vi "对ROI进行分析-修改中.vi"() -> ()   [LabVIEW 2018]
uses:
  <vilib>/vision/NI_Vision_Development_Module.lvlib
panel:
  in  "Pixel Measurements":T1=[0, 1, 2, 3, 42, 8, 9, 10, 11, 4, 5, 6, 7] items=["Center of Mass X", "Center of Mass Y", "First Pixel X", "First Pixel Y", "Bounding Rect Left", "Bounding Rect Top", "Bounding Rect Right", "Bounding Rect Bottom", "Max Feret Diameter Start X", "Max Feret Diameter Start Y", "Max Feret Diameter End X", "Max Feret Diameter End Y", "Max Horiz. Segment Length Left", "Max Horiz. Segment Length Right", "Max Horiz. Segment Length Row", "-", "Bounding Rect Width", "Bounding Rect Height", "Bounding Rect Diagonal", "Perimeter", "Convex Hull Perimeter", "Holes' Perimeter", "Max Feret Diameter", "Equivalent Ellipse Major Axis", "Equivalent Ellipse Minor Axis", "Equivalent Ellipse Minor Axis (Feret)", "Equivalent Rect Long Side", "Equivalent Rect Short Side", "Equivalent Rect Diagonal", "Equivalent Rect Short Side (Feret)", "Average Horiz. Segment Length", "Average Vert. Segment Length", "Hydraulic Radius", "Waddel Disk Diameter", "-", "Area", "Holes' Area", "Particle & Holes' Area", "Convex Hull Area", "Image Area", "-", "Number of Holes", "Number of Horiz. Segments", "Number of Vert. Segments", "-", "Orientation", "Max Feret Diameter Orientation", "-", "% Area/Image Area", "% Area/(Particle & Holes' Area)", "Ratio of Equivalent Ellipse Axes", "Ratio of Equivalent Rect Sides", "-", "Elongation Factor", "Compactness Factor", "Heywood Circularity Factor", "Type Factor", "-", "Sum X", "Sum Y", "Sum XX", "Sum XY", "Sum YY", "Sum XXX", "Sum XXY", "Sum XYY", "Sum YYY", "-", "Moment of Inertia XX", "Moment of Inertia XY", "Moment of Inertia YY", "Moment of Inertia XXX", "Moment of Inertia XXY", "Moment of Inertia XYY", "Moment of Inertia YYY", "Norm. Moment of Inertia XX", "Norm. Moment of Inertia XY", "Norm. Moment of Inertia YY", "Norm. Moment of Inertia XXX", "Norm. Moment of Inertia XXY", "Norm. Moment of Inertia XYY", "Norm. Moment of Inertia YYY", "Hu Moment 1", "Hu Moment 2", "Hu Moment 3", "Hu Moment 4", "Hu Moment 5", "Hu Moment 6", "Hu Moment 7"]
  in  "Selection Values":T3(array[cluster]) {"Measurement Parameter" items=["Center of Mass X", "Center of Mass Y", "First Pixel X", "First Pixel Y", "Bounding Rect Left", "Bounding Rect Top", "Bounding Rect Right", "Bounding Rect Bottom", "Max Feret Diameter Start X", "Max Feret Diameter Start Y", "Max Feret Diameter End X", "Max Feret Diameter End Y", "Max Horiz. Segment Length Left", "Max Horiz. Segment Length Right", "Max Horiz. Segment Length Row", "-", "Bounding Rect Width", "Bounding Rect Height", "Bounding Rect Diagonal", "Perimeter", "Convex Hull Perimeter", "Holes' Perimeter", "Max Feret Diameter", "Equivalent Ellipse Major Axis", "Equivalent Ellipse Minor Axis", "Equivalent Ellipse Minor Axis (Feret)", "Equivalent Rect Long Side", "Equivalent Rect Short Side", "Equivalent Rect Diagonal", "Equivalent Rect Short Side (Feret)", "Average Horiz. Segment Length", "Average Vert. Segment Length", "Hydraulic Radius", "Waddel Disk Diameter", "-", "Area", "Holes' Area", "Particle & Holes' Area", "Convex Hull Area", "Image Area", "-", "Number of Holes", "Number of Horiz. Segments", "Number of Vert. Segments", "-", "Orientation", "Max Feret Diameter Orientation", "-", "% Area/Image Area", "% Area/(Particle & Holes' Area)", "Ratio of Equivalent Ellipse Axes", "Ratio of Equivalent Rect Sides", "-", "Elongation Factor", "Compactness Factor", "Heywood Circularity Factor", "Type Factor", "-", "Sum X", "Sum Y", "Sum XX", "Sum XY", "Sum YY", "Sum XXX", "Sum XXY", "Sum XYY", "Sum YYY", "-", "Moment of Inertia XX", "Moment of Inertia XY", "Moment of Inertia YY", "Moment of Inertia XXX", "Moment of Inertia XXY", "Moment of Inertia XYY", "Moment of Inertia YYY", "Norm. Moment of Inertia XX", "Norm. Moment of Inertia XY", "Norm. Moment of Inertia YY", "Norm. Moment of Inertia XXX", "Norm. Moment of Inertia XXY", "Norm. Moment of Inertia XYY", "Norm. Moment of Inertia YYY", "Hu Moment 1", "Hu Moment 2", "Hu Moment 3", "Hu Moment 4", "Hu Moment 5", "Hu Moment 6", "Hu Moment 7"]; "Range Lower Value" format="%.2f"; "Range Upper Value" format="%.2f"}
  in  "Tab Control":T4
  out "原图":T5(plugin-control) caption="Original Image"
  out "阈值处理":T5(plugin-control) caption="Threshold Image"
  out "面积筛选":T5(plugin-control) caption="Reject Border and Fill Holes"
  out "缺陷统计":T5(plugin-control) caption="Filter Out Non Circles and Overlay Particle Area"
  in  "Stop":bool
  out "Particle Measurements (Pixels)":dbl[][](array[numeric]) format="%.2f"
  in  "Threshold":cluster{"Lower\nValue":sgl, "Upper\nValue":sgl}={"Lower\nValue"=128.0, "Upper\nValue"=255.0}
  in  "Overlay Type":u16[](array[ring])=[2, 1, 3, 0] items=["Rectangle", "Numbers", "Points", "Lines"]
  in  "Color":u32[](array[colorbox])=[3381759, 16776770, 16777225, 6618880]
  # "质心坐标\n\n矩形框左上右下坐标\n\n矩形宽高\n\n周长\n\n等效椭圆长边 短边"
  # "质心\n数量\n费雷特直径\n外接矩形"
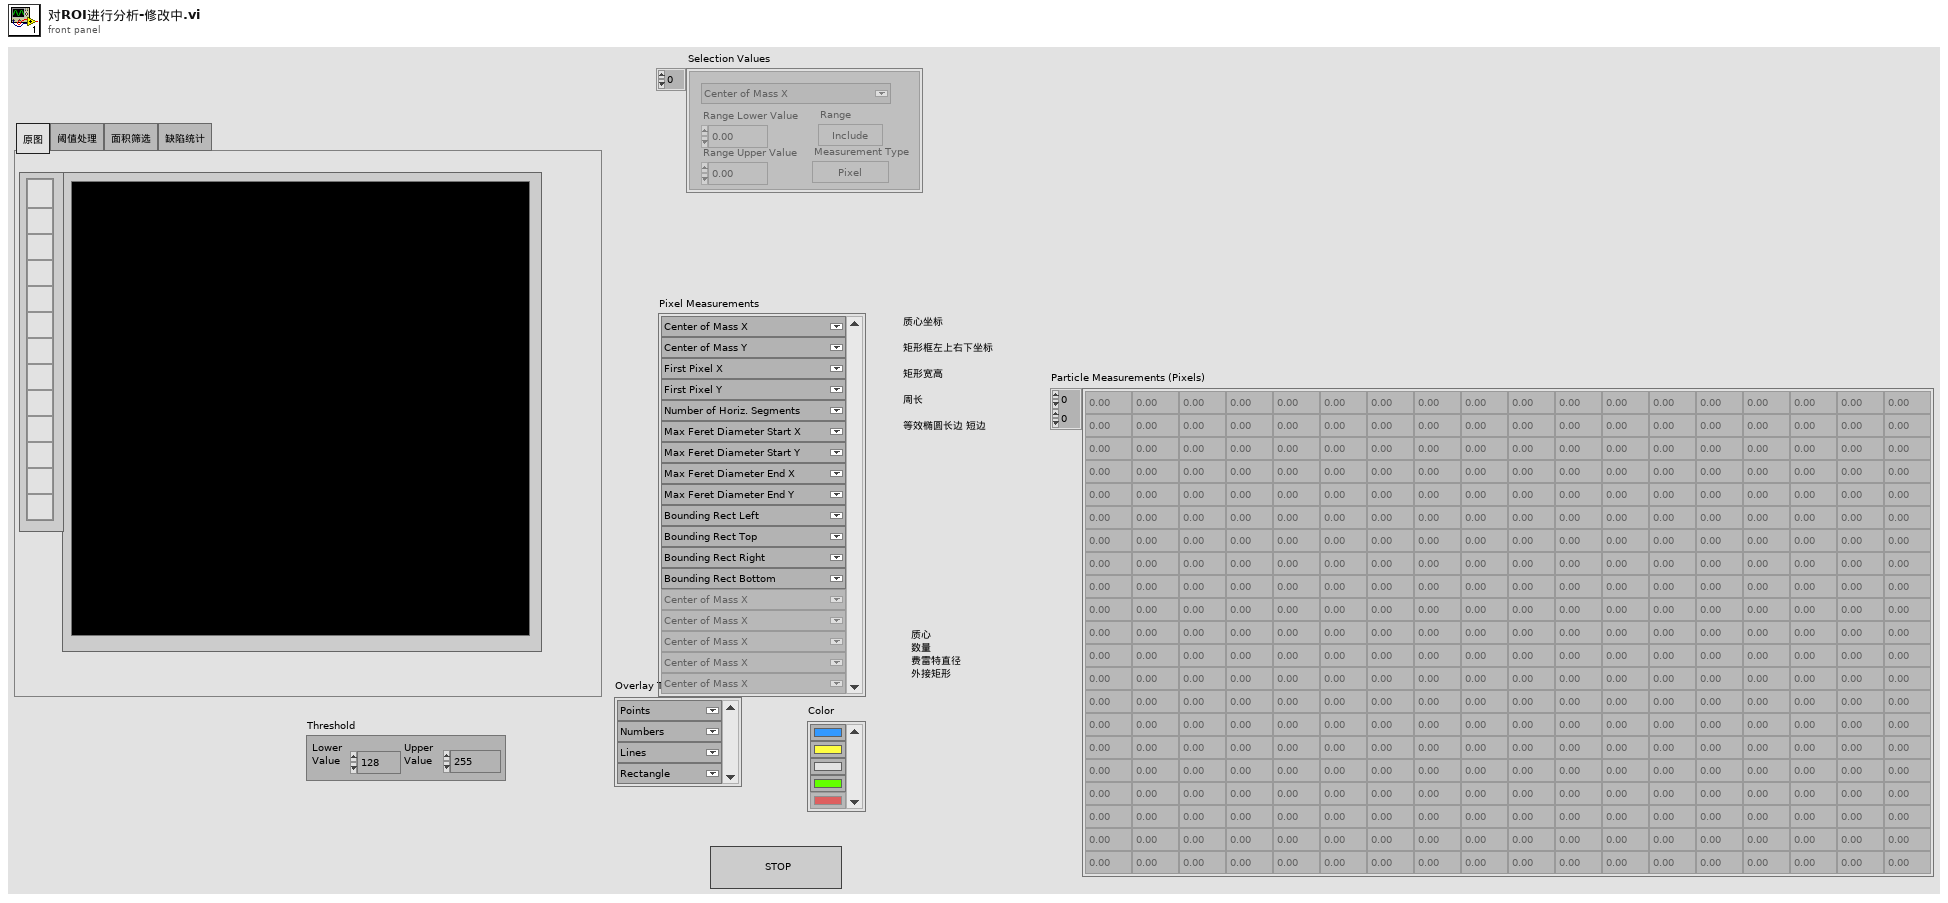
[diagram p1: front panel]
types:
  T1 = typedef "控件 2.ctl" = T2[]
  T2 = typedef "Particle Parameters" = i32
  T3 = cluster{"Measurement Parameter":T2, "Range Lower Value":dbl, "Range Upper Value":dbl, "Range":bool, "Measurement Type":bool}[]
  T4 = typedef "控件 1.ctl" = enum32{"原图", "阈值处理", "面积筛选", "缺陷统计"}
  T5 = typedef "IMAQ Image.ctl" = refnum<image>
  T6 = typedef "Image Type" = u32
  T7 = cluster{"Threshold":cluster{"Lower\nValue":sgl, "Upper\nValue":sgl}, "Pixel Measurements":T1, "Overlay Type":u16[], "Color":u32[]}
  T8 = cluster{"Desired Font (Application)":enum16{"User-specified Font", "Application Font", "System Font", "Dialog Font"}, "[User-specified Font]":cluster{"Font Name":string, "Size":i16, "Strikeout?":bool, "Italic?":bool, "Underline?":bool, "Outline?":bool, "Shadow?":bool, "Bold?":bool, "Rotation Angle":dbl}, "Horizontal Alignment":i16, "Vertical Alignment":i16}
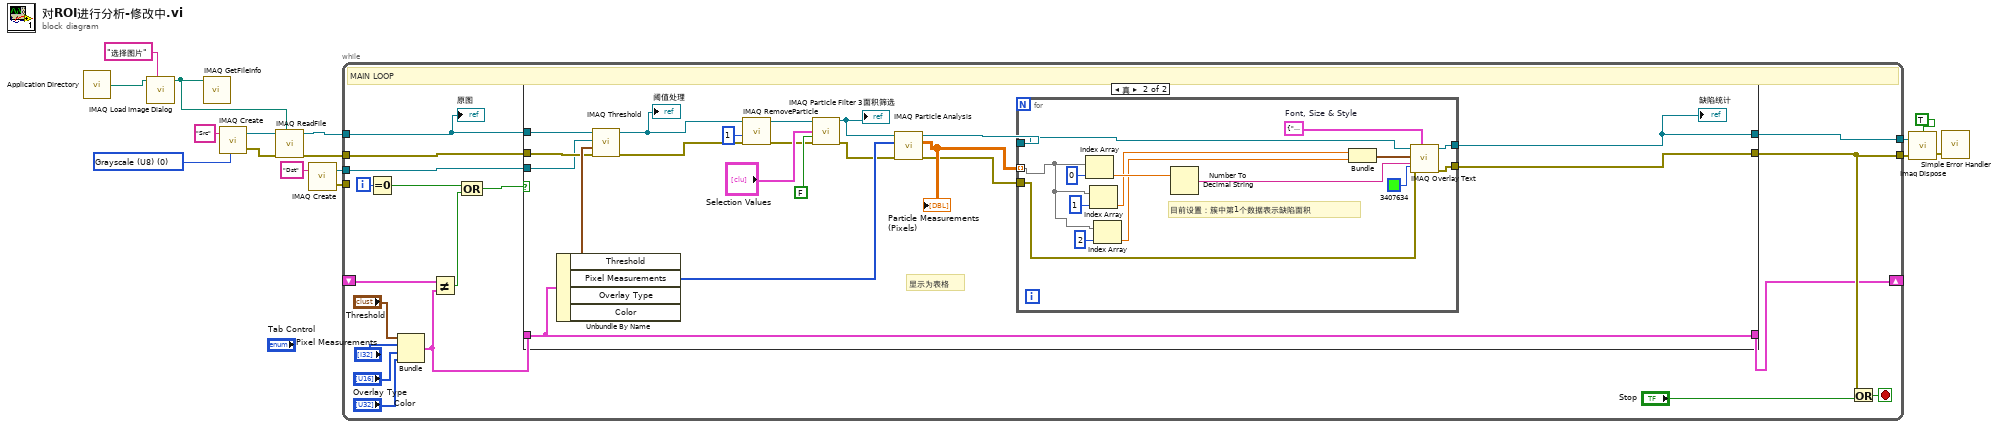
[diagram p0: block diagram]
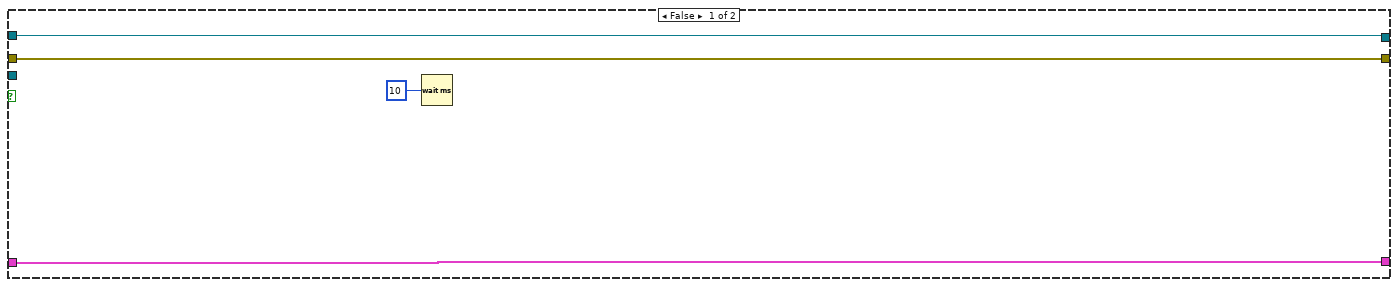
[diagram p2: hidden frame]
diagram:
  w2 = T6 0 items=["Grayscale (U8)", "Grayscale (I16)", "Grayscale (SGL)", "Complex (CSG)", "RGB (U32)", "HSL (U32)", "RGB (U64)", "Grayscale (U16)"] ("Image Type")
  n1 = call <vilib>:"Application Directory.vi"() -> ("Application Directory"=w4:path)
  n2 = call "IMAQ Load Image Dialog"("Prompt"="选择图片" ("prompt"), "Start Path"=w4) -> ("Path"=w3:path)  [unwired: 7 in, 2 out]
  n3 = call "IMAQ GetFileInfo"("File Path"=w3) -> ()  [unwired: 4 in, 7 out]
  n4 = call "IMAQ Create"("Image Name"="Src", "Image Type"=w2) -> ("New Image"=w15:T5, "error out"=w14:errorcluster)  [unwired: 3 in]
  n5 = call "IMAQ ReadFile"("File Path"=w3, "error in (no error)"=w14, "Image"=w15) -> ("error out"=w10:errorcluster, "Image Out"=w9:T5)  [unwired: 4 in, 3 out]
  n6 = call "IMAQ Create"("Image Name"="Dst") -> ("New Image"=w7:T5, "error out"=w6:errorcluster)  [unwired: 4 in]
  n7 = while "MAIN LOOP" {
    tunnel: w9 -> [w19]
    tunnel: w10 -> [w22]
    tunnel: [w32] -> w13
    shift-right: [w29] -> _
    shift-left: _ -> [w27]
    tunnel: w7 -> [w23]
    tunnel: w6 -> [_]
    tunnel: [w18] -> w1
    i -> [w31]
    stop <- w33 stop-if-true
    # "MAIN LOOP"
    n8 = Equal To 0?(x=w31) -> (x = 0?=w28:bool)
    n9 = Bundle("Threshold"="Threshold", "Pixel Measurements"="Pixel Measurements", "Overlay Type"="Overlay Type", "Color"="Color") -> (w25:T7)  [unwired: 1 in]
    n10 = Not Equal?(x=w27, y=w25) -> (x != y?=w26:bool)
    n11 = Compound Arithmetic op=OR(w28, w26) -> (w30:bool)
    n12 = case shown="真" w30 {
      tunnel: w22 -> [w38 w56]
      tunnel: w19 -> [w35 w55]
      tunnel: [w35 w40] -> w18
      tunnel: [w38 w39] -> w32
      tunnel: [w37 w58] -> w29
      tunnel: w25 -> [w37 w58]
      tunnel: w23 -> [_ w53]
      frame False {
        n13 = Wait (ms)(milliseconds to wait=u32 10) -> ()  [unwired: 1 out]
      }
      frame True {
        # "显示为表格"
        n14 = Unbundle By Name(w58) -> ("Threshold"=w57:cluster{"Lower\nValue":sgl, "Upper\nValue":sgl}, "Pixel Measurements"=w54:T1)  [unwired: 2 out]
        n15 = call "IMAQ Threshold"("error in (no error)"=w56, "Range"=w57, "Image Dst"=w53, "Image Src"=w55) -> ("error out"=w47:errorcluster, "Image Dst Out"=w51:T5)  [unwired: 2 in, 4 out]
        "阈值处理" <- w51
        n16 = call "IMAQ RemoveParticle"("error in (no error)"=w47, "Number of Erosion"=1, "Image Src"=w51) -> ("error out"=w46:errorcluster, "Image Dst Out"=w50:T5)  [unwired: 7 in]
        n17 = call "IMAQ Particle Filter 3"("Image Src"=w50, "Selection Values"="Selection Values", "Keep/Remove Particles (F)"=FALSE, "error in (no error)"=w46) -> ("Image Dst Out"=w44:T5, "error out"=w45:errorcluster)  [unwired: 9 in, 1 out]
        "面积筛选" <- w44
        n18 = call "IMAQ Particle Analysis"("error in (no error)"=w45, "Pixel Measurements"=w54, "Image"=w44) -> ("error out"=w41:errorcluster, "Particle Measurements (Pixels)"=w43:dbl[][], "Image Out (duplicate)"=w42:T5)  [unwired: 3 in, 3 out]
        "Particle Measurements (Pixels)" <- w43
        n19 = for {
          tunnel: w41 -> [w73]
          tunnel: [w72] -> w39
          tunnel: [w71] -> w40
          tunnel: w42 -> [w69]
          tunnel: w43 -> [w61] mode=indexing
          w68 = T8 {"Desired Font (Application)"=enum."Application Font", "[User-specified Font]"={"Font Name"="", "Size"=12, "Strikeout?"=FALSE, "Italic?"=FALSE, "Underline?"=FALSE, "Outline?"=FALSE, "Shadow?"=FALSE, "Bold?"=FALSE, "Rotation Angle"=0.0}, "Horizontal Alignment"=0, "Vertical Alignment"=0}  # Font, Size & Style
          # "目前设置：簇中第1个数据表示缺陷面积"
          n20 = Index Array(array=w61, index=0 ("索引")) -> (element=w66:dbl)
          n21 = Index Array(array=w61, index=1 ("索引")) -> (element=w63:dbl)
          n22 = Index Array(array=w61, index=2 ("索引")) -> (element=w60:dbl)
          n23 = Number To Decimal String(number=w66) -> (decimal integer string=w67:string)  [unwired: 1 in]
          n24 = Bundle("Numeric"=w63, "Numeric"=w60) -> (w59:cluster{"Numeric":dbl, "Numeric":dbl})  [unwired: 1 in]
          n25 = call "IMAQ Overlay Text"("Text Color (black)"=u32 3407634, "Font, Size & Style"=w68, "error in (no error)"=w73, "String"=w67, "Origin"=w59, "Image"=w69) -> ("error out"=w72:errorcluster, "Image Out"=w71:T5)  [unwired: 4 in]
        }
        "缺陷统计" <- w40
      }
    }
    n26 = Or(x=w32, y="Stop") -> (x .or. y?=w33:bool)
    "原图" <- w19
  }
  n27 = call "Imaq Dispose"("All Images? (No)"=TRUE, "Image"=w1, "error in (no error)"=w13) -> ("error out"=w12:errorcluster)  [unwired: 3 in]
  n28 = call <vilib>:"Simple Error Handler.vi"("error in (no error)"=w12) -> ()  [unwired: 4 in, 5 out]
